vi "Get last selected item.vi"(8 "error in (no error)":errorcluster, 11 "Pool":T1[](array[typedef])=[{"index"=0, "state"=enum."unused"}, {"index"=1, "state"=enum."unused"}, {"index"=2, "state"=enum."unused"}, {"index"=3, "state"=enum."unused"}, {"index"=4, "state"=enum."unused"}, {"index"=5, "state"=enum."unused"}]) -> (0 "error out":errorcluster, 1 "index of last selected item":i32, 2 "T = selected item was found":bool, 3 "Last selected item":T1)   [LabVIEW 2021, in "Numeric Utilities.lvlib"]
uses:
  Numeric Utilities.lvlib
  cluster-touched index.ctl
  index state enum.ctl
panel:
  # "Development\ncontrols/indicators useful for development and testing, but which are not outputs of the VI"
  # "Input\nInputs to the VI"
  # "Output\nOutputs of the VI"
  # "Description\n\nBlank VI with error handling case. \n\nSummarize the use of this VI in this space."
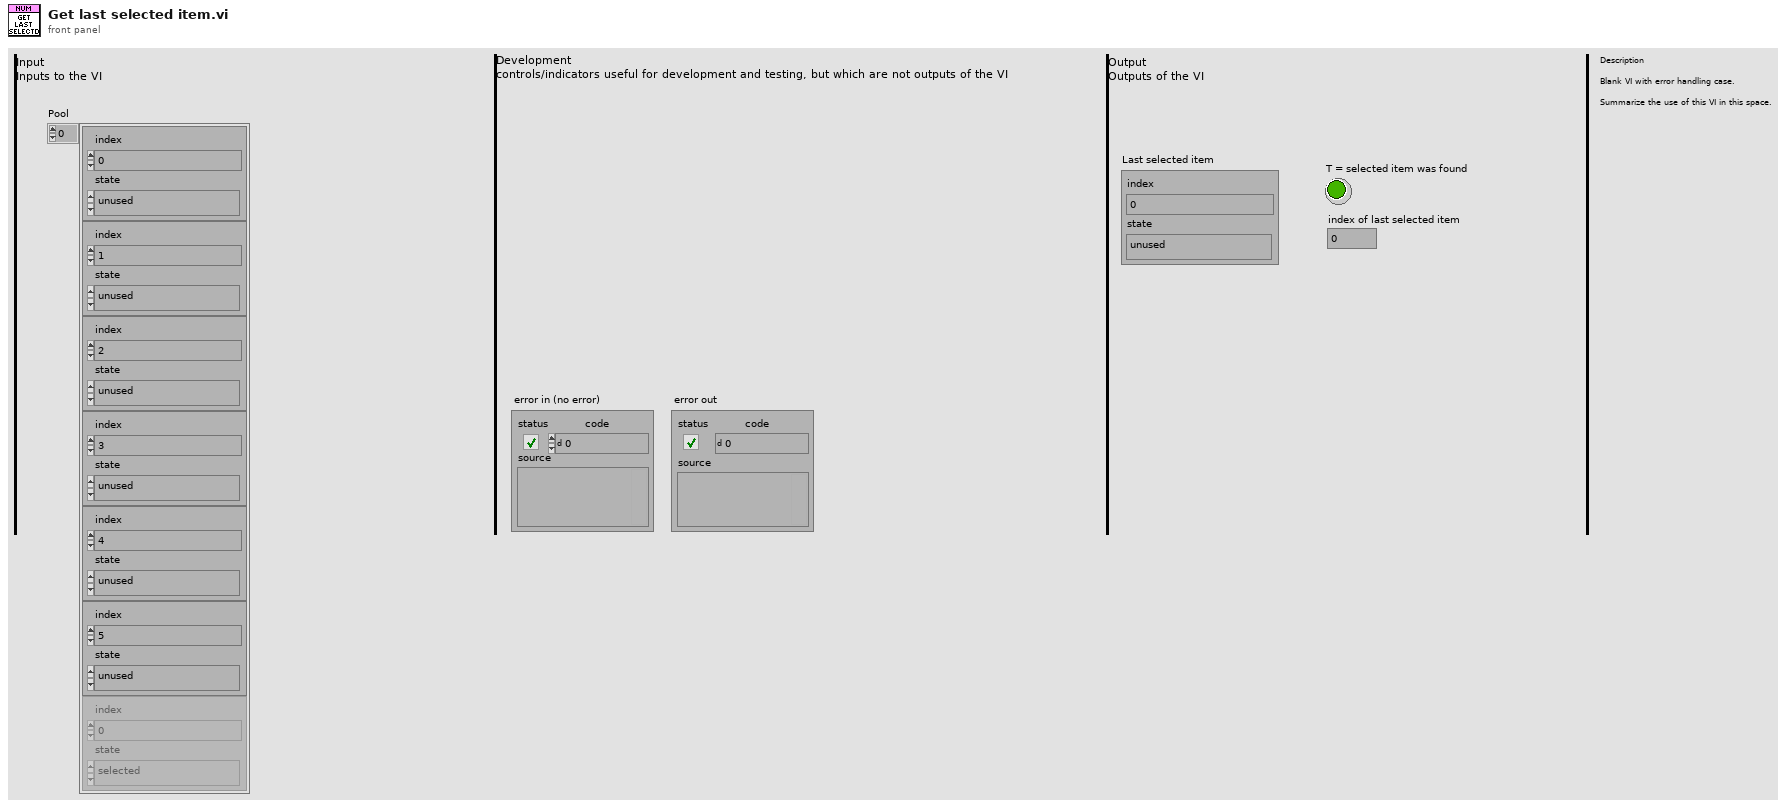
[diagram p1: front panel]
types:
  T1 = typedef "Numeric Utilities.lvlib/cluster-touched index.ctl" = cluster{"index":i32, "state":T2}
  T2 = typedef "Numeric Utilities.lvlib/index state enum.ctl" = enum16{"unused", "selected", "exhausted"}
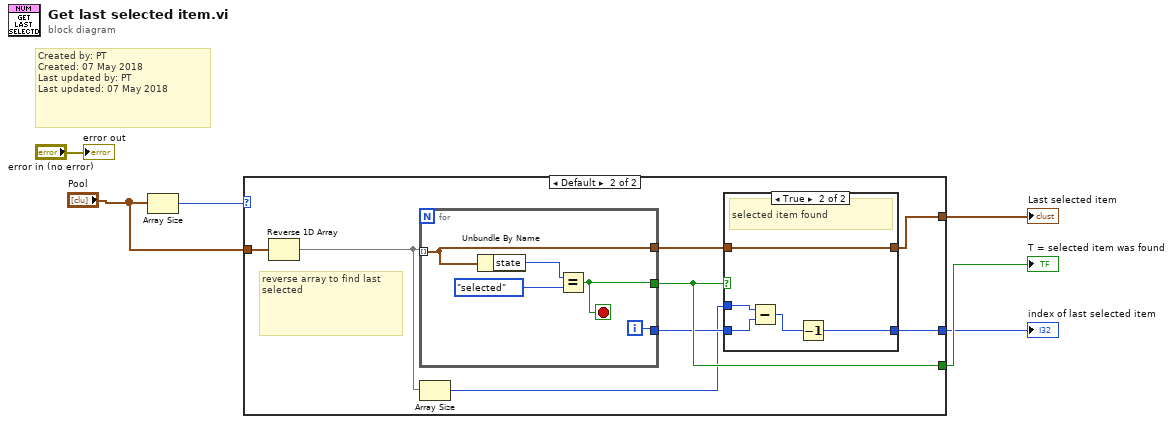
[diagram p0: block diagram]
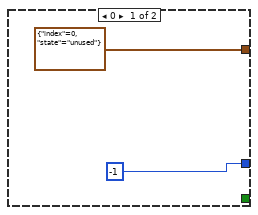
[diagram p2: hidden frame]
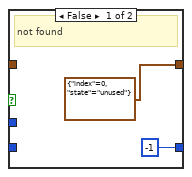
[diagram p3: hidden frame]
diagram:
  # "Created by: PT\nCreated: 07 May 2018\nLast updated by: PT\nLast updated: 07 May 2018"
  n1 = Array Size(array="Pool") -> (size(s)=w4:i32)
  n2 = case shown="Default" w4 {
    tunnel: "Pool" -> [_ w16]
    tunnel: [_ w15] -> w3
    tunnel: [T1 {"index"=0, "state"=enum."unused"} w13] -> w2
    tunnel: [-1 w11] -> w1
    frame 0 {
    }
    frame Default {
      # "reverse array to find last selected"
      n3 = Reverse 1D Array(array=w16) -> (reversed array=w10:T1[])
      n4 = for {
        tunnel: w10 -> [w25] mode=indexing
        tunnel: [w26] -> w15
        tunnel: [w25] -> w14
        tunnel: [w24] -> w12
        i -> [w24]
        stop <- w26 stop-if-true
        n5 = Unbundle By Name(w25) -> ("state"=w28:T2)
        n6 = Equal?(x=w28, y=index_state_enum."selected") -> (x = y?=w26:bool)
      }
      n7 = Array Size(array=w10) -> (size(s)=w9:i32)
      n8 = case shown="True" w15 {
        tunnel: w14 -> [_ w23]
        tunnel: [T1 {"index"=0, "state"=enum."unused"} w23] -> w13
        tunnel: w12 -> [_ w21]
        tunnel: [-1 w19] -> w11
        tunnel: w9 -> [_ w22]
        frame False {
          # "not found"
        }
        frame True {
          # "selected item found"
          n9 = Subtract(x=w22, y=w21) -> (x-y=w20:i32)
          n10 = Decrement(x=w20) -> (x-1=w19:i32)
        }
      }
    }
  }
  "T = selected item was found" <- w3
  "Last selected item" <- w2
  "index of last selected item" <- w1
  "error out" <- "error in (no error)"
